vi "[Advanced] Modify an Existing Package File (Unpack Modify Pack).vi"() -> ()   [LabVIEW 2014]
doc: "This example shows how to unpack an existing package, modify the package data/metadata, and pack the modifications into a new package."
uses:
  _support/package attributes.ctl
  <vilib>/Utility/sysdir.llb/System Directory Type.ctl
  NIPM_API.lvlib
panel:
  out "Unpacked folderpath":path
  out "Modified package filepath":path
  in  "Modified Package Attributes":T1={"Package Name"="", "Display name"="", "Version"="", "Display version"="", "Synopsis"="", "Description"="", "Maintainer"="", "Maintainer email address"="", "Category"="", "Homepage"="", "Release notes"="", "Depends"=[], "Recommends"=[], "Suggests"=[], "Conflicts"=[], "Provides"=[], "Replaces"=[], "Supplements"=[], "Enhances"=[], "Product"=FALSE, "User visible"=FALSE, "Installed size (KB)"=0, "Package filesize (bytes)"=0, "Architecture"="", "Agent"="file", "MD5Checksum"=""}
  in  "Pack modified package":bool
  in  "Unpack":bool
  in  "Destination folder for modified package":path
  in  "Original package filepath":path
  out "Original Package Attributes":T1={"Package Name"="", "Display name"="", "Version"="", "Display version"="", "Synopsis"="", "Description"="", "Maintainer"="", "Maintainer email address"="", "Category"="", "Homepage"="", "Release notes"="", "Depends"=[], "Recommends"=[], "Suggests"=[], "Conflicts"=[], "Provides"=[], "Replaces"=[], "Supplements"=[], "Enhances"=[], "Product"=FALSE, "User visible"=FALSE, "Installed size (KB)"=0, "Package filesize (bytes)"=0, "Architecture"="", "Agent"="file", "MD5Checksum"=""}
  # "1. Choose the original package you want to modify.\n2. Click the Unpack button to unpack the package to a temporary directory.\n3. View the package attributes."
  # "4. Modify the desired package attributes below.  These modifications will be passed to the controls file when you click the Pack button in Step 6.\n\nYou can also navigate to the \"Unpacked folderpath\" to modify the data folder contents and the instructions file manually."
  # "5. Choose the destination folder for your modified package.\n6. Click the Pack button.\n7. View the filepath for your modified package."
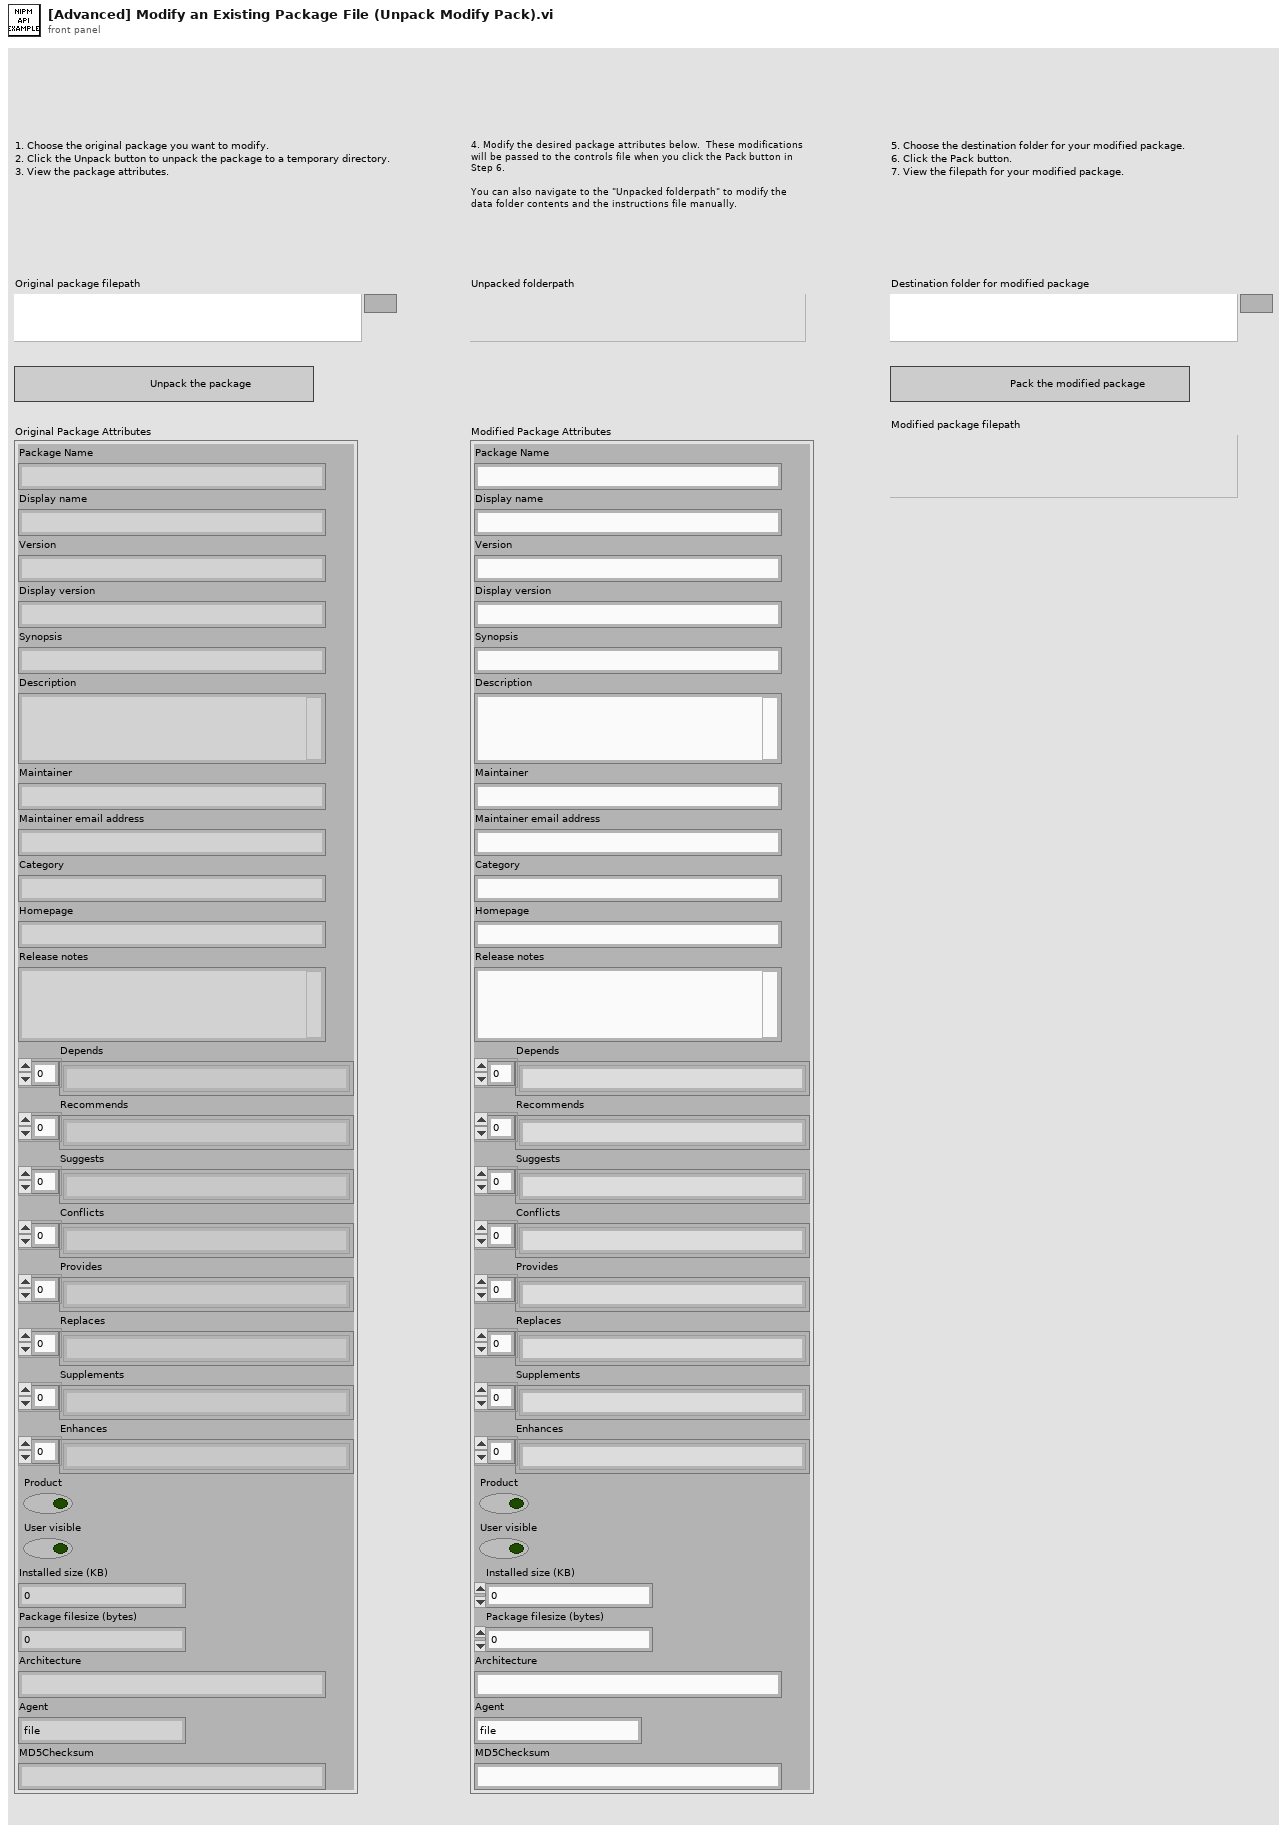
[diagram p1: front panel]
types:
  T1 = typedef "NIPM_API.lvlib/package attributes.ctl" = cluster{"Package Name":string, "Display name":string, "Version":string, "Display version":string, "Synopsis":string, "Description":string, "Maintainer":string, "Maintainer email address":string, "Category":string, "Homepage":string, "Release notes":string, "Depends":string[], "Recommends":string[], "Suggests":string[], "Conflicts":string[], "Provides":string[], "Replaces":string[], "Supplements":string[], "Enhances":string[], "Product":bool, "User visible":bool, "Installed size (KB)":u64, "Package filesize (bytes)":u64, "Architecture":string, "Agent":string, "MD5Checksum":string}
  T2 = typedef "System Directory Type.ctl" = i32
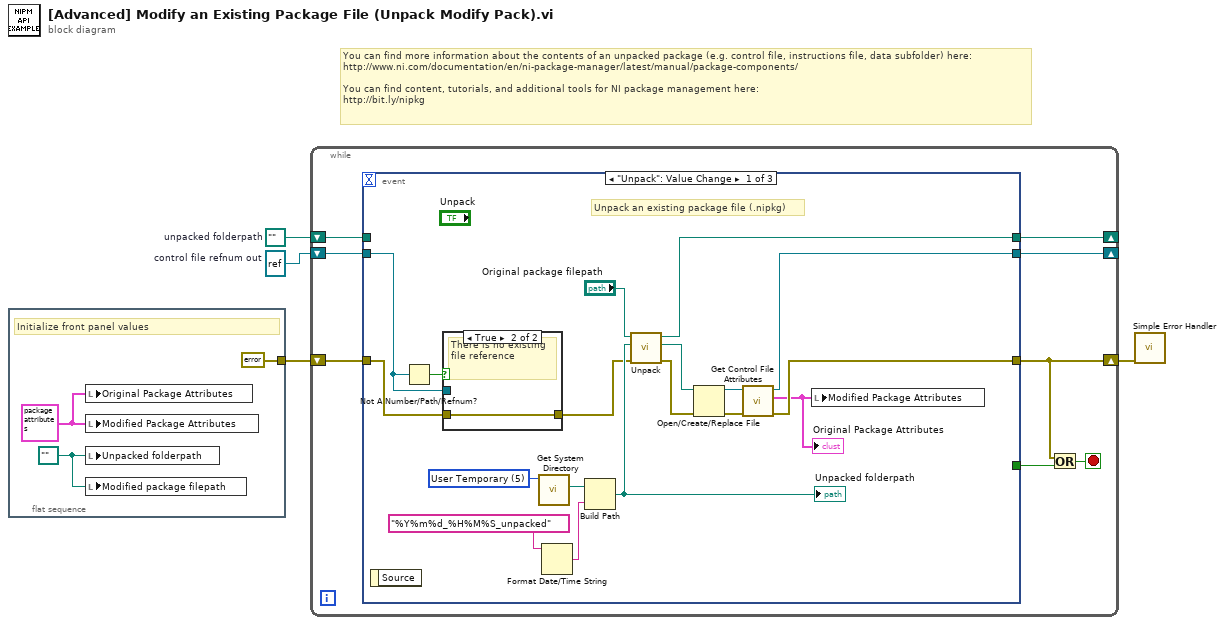
[diagram p0: block diagram]
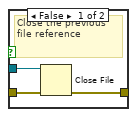
[diagram p2: hidden frame]
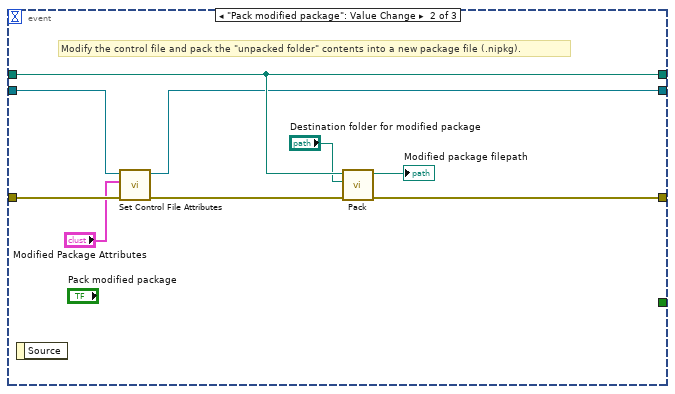
[diagram p3: hidden frame]
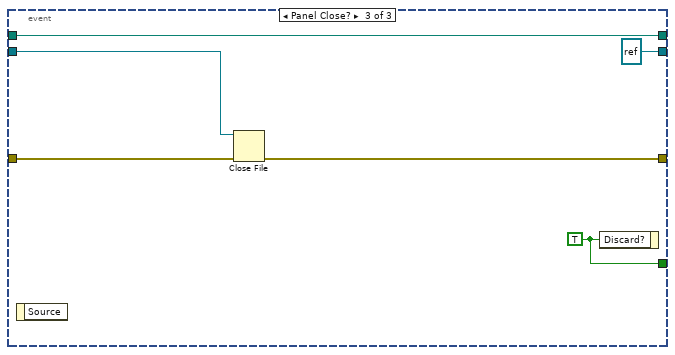
[diagram p4: hidden frame]
diagram:
  w3 = refnum<file> refnum  # control file refnum out
  w4 = path ""  # unpacked folderpath
  # "You can find more information about the contents of an unpacked package (e.g. control file, instructions file, data subfolder) here:\nhttp://www.ni.com/documentation/en/ni-package-manager/latest/manual/package-components/\n\nYou can find content, tutorials, and additional tools for NI package management here:\nhttp://bit.ly/nipkg"
  n1 = flat-sequence {
    tunnel: [errorcluster {"status"=FALSE, "code"=0, "source"=""} ("error out")] -> w2
    frame #0 {
      w6 = path "" ("Modified package filepath")
      w7 = T1 {"Package Name"="", "Display name"="", "Version"="", "Display version"="", "Synopsis"="", "Description"="", "Maintainer"="", "Maintainer email address"="", "Category"="", "Homepage"="", "Release notes"="", "Depends"=[], "Recommends"=[], "Suggests"=[], "Conflicts"=[], "Provides"=[], "Replaces"=[], "Supplements"=[], "Enhances"=[], "Product"=FALSE, "User visible"=FALSE, "Installed size (KB)"=0, "Package filesize (bytes)"=0, "Architecture"="", "Agent"="file", "MD5Checksum"=""} ("Original Package Attributes")
      # "Initialize front panel values"
      n2 = local write "Original Package Attributes"(w7) -> ()
      n3 = local write "Modified Package Attributes"(w7) -> ()
      n4 = local write "Unpacked folderpath"(w6) -> ()
      n5 = local write "Modified package filepath"(w6) -> ()
    }
  }
  n6 = while {
    shift-right: [w15] -> _
    shift-left: w4 -> [w14]
    shift-right: [w10] -> w1
    shift-left: w2 -> [w13]
    shift-right: [w11] -> _
    shift-left: w3 -> [w12]
    stop <- w8 stop-if-true
    n7 = event shown="[0] \"Unpack\": Value Change" {
      selector: _ -> [_ _ _]
      dyn-events: _ -> [_ _ _]
      timeout: _ -> [_ _ _]
      tunnel: [w29 w46 w52] -> w15
      tunnel: w14 -> [_ w46 w52]
      tunnel: [w27 w43 w49] -> w10
      tunnel: w13 -> [w18 w42 w51]
      tunnel: w12 -> [w16 w40 w48]
      tunnel: [w26 w38 refnum<file> refnum ("control file refnum out")] -> w11
      tunnel: [_ _ w50] -> w9
      event "Unpack": Value Change {
        w24 = T2 5 items=["User Home"=0, "User Desktop"=1, "User Documents"=2, "User Application Data"=3, "User Preferences"=4, "User Temporary"=5, "Public Documents"=6, "Public Application Data"=7, "Public Preferences"=8, "Public Cache"=13, "System Core Libraries"=9, "System Installed Libraries"=10, "Application Files"=11, "Boot Volume Root"=12] ("system directory type")
        # "Unpack an existing package file (.nipkg)"
        n8 = event-data() -> ()  [unwired: 1 in, 1 out]
        n9 = Not A Number/Path/Refnum?(number/path/refnum=w16) -> (NaN/Path/Refnum?=w19:bool)
        n10 = case shown="True" w19 {
          tunnel: w18 -> [w36 w37]
          tunnel: [w35 w37] -> w17
          tunnel: w16 -> [w34 _]
          frame False {
            # "Close the previous file reference"
            n11 = Close File(refnum=w34, error in=w36) -> (error out=w35:errorcluster)  [unwired: 1 out]
          }
          frame True {
            # "There is no existing file reference"
          }
        }
        n12 = call <vilib>:"Get System Directory.vi"("system directory type"=w24) -> ("system directory"=w23:path)  [unwired: 10 in]
        n13 = Format Date/Time String(time format string (%c)="%Y%m%d_%H%M%S_unpacked") -> (date/time string=w21:string)  [unwired: 2 in]
        n14 = Build Path(base path=w23, name or relative path=w21) -> (appended path=w20:path)
        "Unpacked folderpath" <- w20
        n15 = call "Unpack.vi"("error in"=w17, "destination folder"=w20, "nipkg filepath"="Original package filepath") -> ("error out"=w28:errorcluster, "control filepath"=w32:path, "unpacked folderpath"=w29:path)  [unwired: 4 in, 2 out]
        n16 = Open/Create/Replace File(file path (use dialog)=w32, error in=w28) -> (refnum out=w31:refnum<file>, error out=w30:errorcluster)  [unwired: 4 in, 1 out]
        n17 = call "Get Control File Attributes.vi"("error in (no error)"=w30, "control file refnum in"=w31) -> ("error out"=w27:errorcluster, "package attributes"=w25:T1, "control file refnum out"=w26:refnum<file>)  [unwired: 7 in]
        "Original Package Attributes" <- w25
        n18 = local write "Modified Package Attributes"(w25) -> ()
      }
      event "Pack modified package": Value Change {
        # "Modify the control file and pack the \"unpacked folder\" contents into a new package file (.nipkg)."
        n19 = event-data() -> ()  [unwired: 1 in, 1 out]
        n20 = call "Set Control File Attributes.vi"("error in (no error)"=w42, "package attributes"="Modified Package Attributes", "control file refnum in"=w40) -> ("error out"=w41:errorcluster, "control file refnum out"=w38:refnum<file>)  [unwired: 7 in]
        n21 = call "Pack.vi"("error in"=w41, "destination folder"="Destination folder for modified package", "source folder"=w46) -> ("error out"=w43:errorcluster, "package filepath"=→"Modified package filepath":path)  [unwired: 7 in]
      }
      event Panel Close? {
        w50 = TRUE ("Discard?")
        n22 = event-data() -> ()  [unwired: 1 in, 1 out]
        n23 = Close File(refnum=w48, error in=w51) -> (error out=w49:errorcluster)  [unwired: 1 out]
        n24 = event-data("Discard?"=w50) -> ()  [unwired: 1 in, 1 out]
      }
    }
    n25 = Or(x=w10, y=w9) -> (x .or. y?=w8:bool)
  }
  n26 = call <vilib>:"Simple Error Handler.vi"("error in (no error)"=w1) -> ()  [unwired: 4 in, 5 out]
